vi "positionerCapture_example.vi"() -> ()   [LabVIEW 2023]
doc: "CONEX - CC Virtual Front Panel:\n\nThis is a sample of an application that can be built with the LabVIEW drivers.\n\nPress HOME / ENABLE in top left of panel to put stage in Ready state for motion."
uses:
  <vilib>/userDefined/High Color/IMAQdx.ctl
  <vilib>/Platform/TimedLoop/XDataNode/timing_clust.ctl
  <vilib>/Platform/TimedLoop/XDataNode/nitl_modes.ctl
  <vilib>/Platform/TimedLoop/XDataNode/wakeup.ctl
  <vilib>/Platform/TimedLoop/XDataNode/XDataNode.xnode
  <vilib>/Platform/TimedLoop/XDataNode/XDNodeRunTimeDep.lvlib
  <vilib>/vision/driver/NI_Vision_Acquisition_Software.lvlib
panel:
  in  "Session In":T1="BW14bits Focused"
  out "Current noUnits":dbl caption="mm" format="%#_6f"
  in  "lambda":dbl caption="nm" format="%#_6f"
  in  "Units":string(combo)="mm"
  in  "Go0":bool
  in  "Zero position":dbl caption="lam" format="%#_6f"
  in  "Tare":bool
  out "Relative position":dbl caption="lam" format="%#_6f"
  in  "Path to save the captures":path
  out "Image":T2(plugin-control)
  in  "(1) Go to:":dbl=1.0 caption="lam"
  out "Title":string
  in  "Set Max":bool
  in  "Set Min":bool
  in  "Max":dbl
  in  "Min":dbl
  in  "Set velocity":bool
  out "Stop cycle":bool=TRUE
  out "Title 2":string
  in  "Cycle":bool
  in  "Go2":bool
  in  "Go1":bool
  in  "(2) Go to:":dbl=1.0 caption="lam"
  in  "-":bool
  in  "+":bool
  in  "Step:":dbl caption="lam" format="%#_6f"
  out "Position History":dbl(graph)=1.5
  in  "Action":bool
  out "Stop polling":bool=TRUE
  out "Controller state description":string="STATUS"
  out "Velocity MAX":dbl=0.4
  out "Controller state":string="33"
  out "Positioner error":string="0000"
  in  "Velocity:":dbl format="%#_6f"
  in  "Exit":bool=TRUE
  out "Target position":dbl
  in  "Exit":bool
  in  "Position glissière":cluster{dbl, dbl}(slide) scale=0.0..25.0
  out "Current position":dbl caption="lam" format="%#_6f"
  # "mm/s"
  # "mm"
  # "Limits:"
  # "mm"
  # "(1)"
  # "(2)"
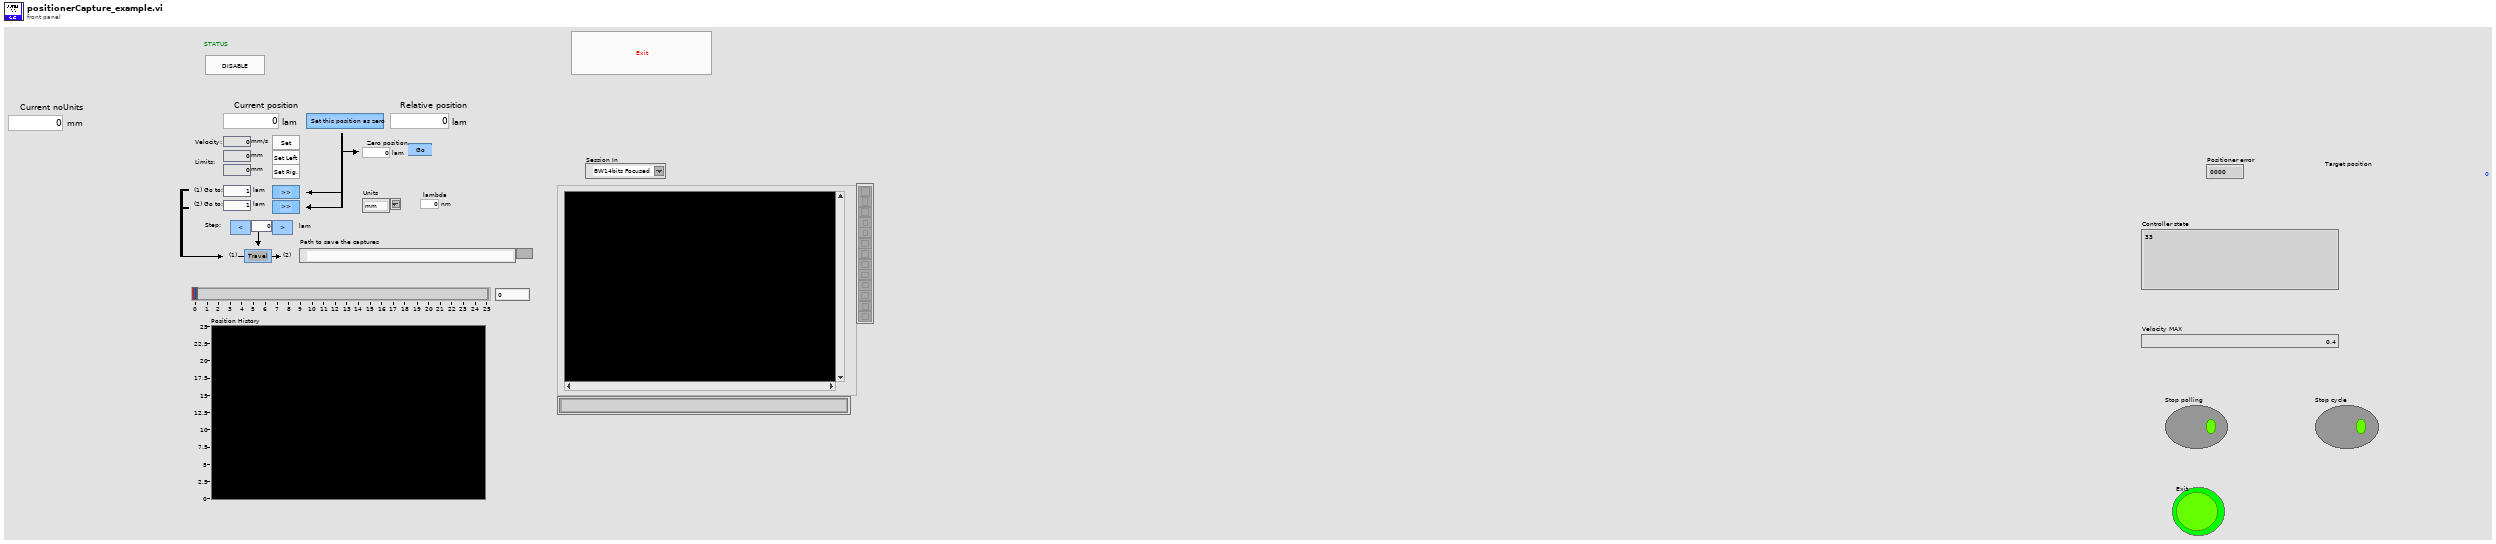
[diagram p1: front panel]
types:
  T1 = typedef "IMAQdx.ctl" = refnum<k21>
  T2 = typedef "IMAQ Image.ctl" = refnum<image>
  T3 = typedef "XDNodeRunTimeDep.lvlib/timing_clust.ctl" = cluster{"Expected End [f-1]":u64, "Actual End [f-1]":u64, "Finished Late? [f-1]":bool, "Expected End [i-1]":u64, "Actual End [i-1]":u64, "Finished Late? [i-1]":bool, "Expected Start [i]":u64, "Actual Start [i]":u64, "Expected Start [f]":u64, "Actual Start [f]":u64, "Source Name":string, "Structure Name":string, "Period":i64, "Deadline":i64, "Offset":i64, "Start":i64, "Priority":i32, "Timeout":i32, "Mode":T4, "Wakeup Reason":T5, "Error":errorcluster, "Source Type":string, "Secondary Source Type":string, "Global End Time":u64, "Global Start Time":u64, "Frame Duration":u64, "Iteration Duration":u64, "Assigned CPU":i32, "I/O Scan Engine Mode":u32}
  T4 = typedef "XDNodeRunTimeDep.lvlib/nitl_modes.ctl" = enum32{"No Change", "Process missed periods, maintain original phase", "Discard missed periods, maintain original phase", "Process missed periods, ignore original phase", "Discard missed periods, ignore original phase"}
  T5 = typedef "XDNodeRunTimeDep.lvlib/wakeup.ctl" = enum32{"Normal", "Aborted", "Asynchronous wakeup", "Timing source error", "Timed loop error", "Timeout"}
  T6 = cluster{"VISA resource name":refnum<visa-resource-name>, "Device name":string, "Controller address":i32, "error":errorcluster}
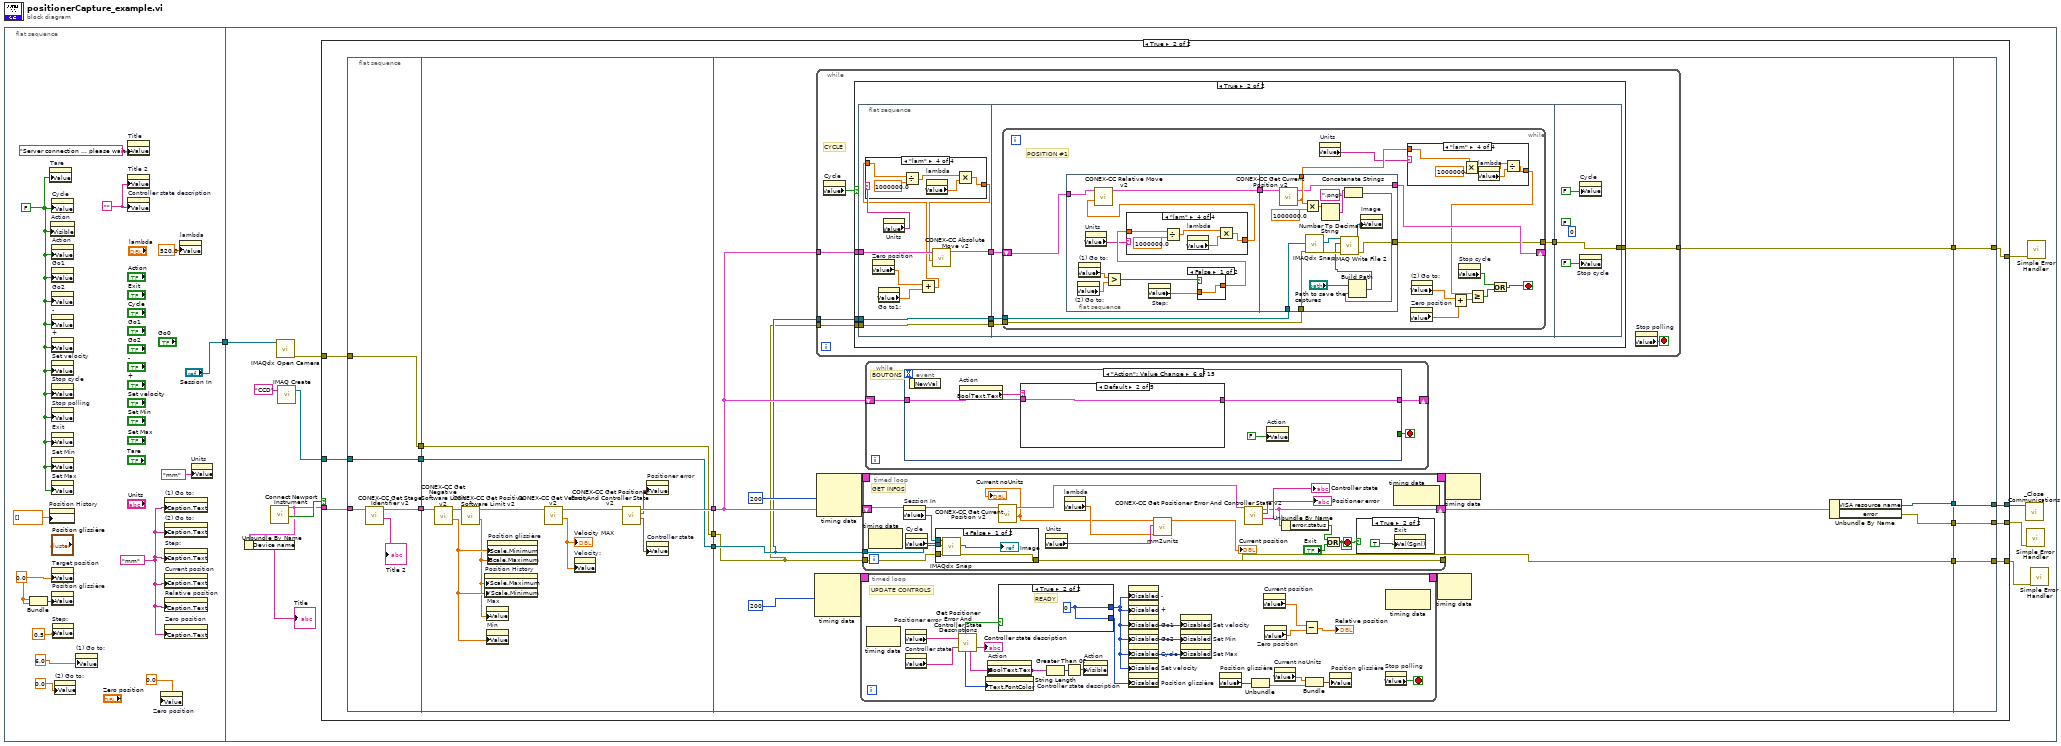
[diagram p0: block diagram]
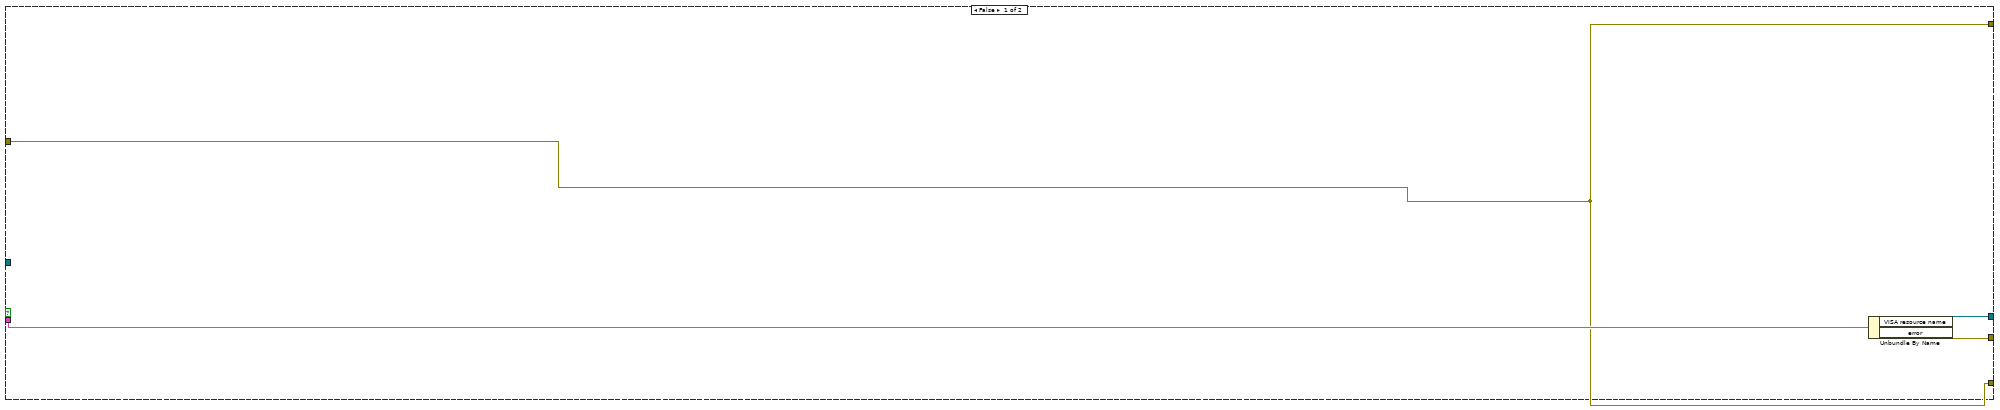
[diagram p2: hidden frame]
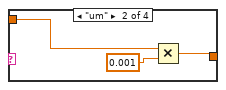
[diagram p5: hidden frame]
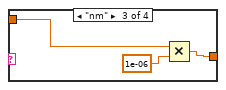
[diagram p6: hidden frame]
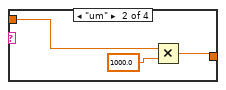
[diagram p8: hidden frame]
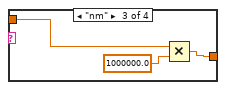
[diagram p9: hidden frame]
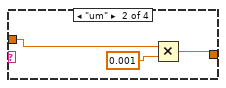
[diagram p11: hidden frame]
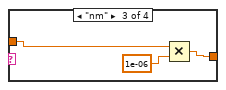
[diagram p12: hidden frame]
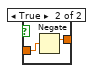
[diagram p13: hidden frame]
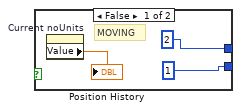
[diagram p14: hidden frame]
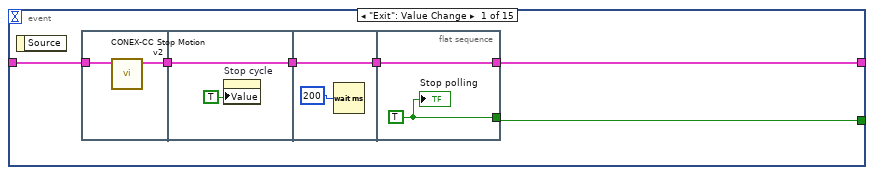
[diagram p15: hidden frame]
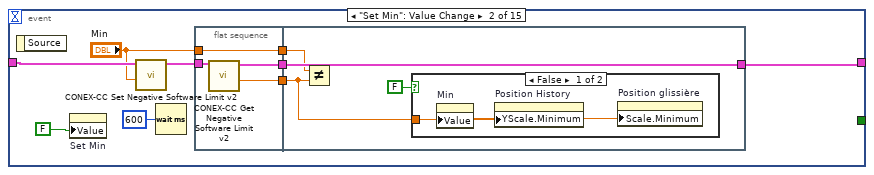
[diagram p16: hidden frame]
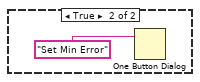
[diagram p17: hidden frame]
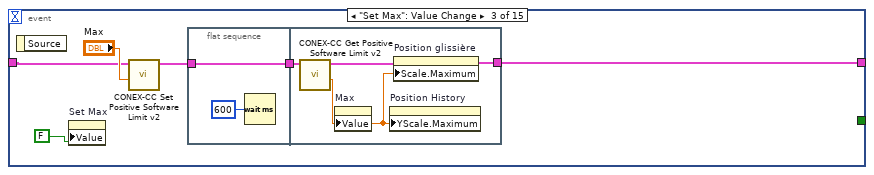
[diagram p18: hidden frame]
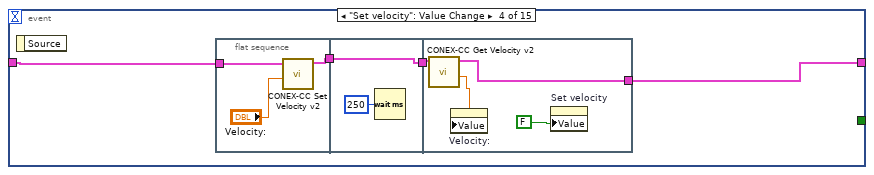
[diagram p19: hidden frame]
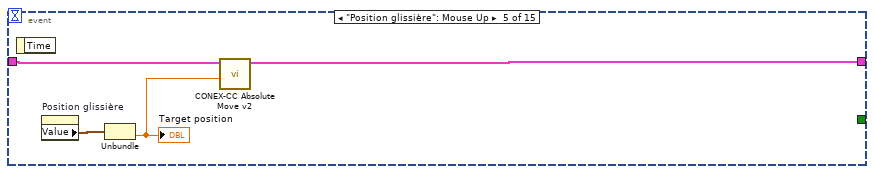
[diagram p20: hidden frame]
diagram:
  n1 = flat-sequence {
    tunnel: ["Session In"] -> w1
    tunnel: w1 -> [w16]
    frame #0 {
      w4 = "mm" ("Units")
      w8 = FALSE
      w14 = 0.0
      w13 = ""
      n2 = Bundle(w14, w14) -> (w15:cluster{dbl, dbl})  [unwired: 1 out]
      n3 = property on="Position History" class="WFChart (strict)"("History Data"=dbl[] [] ("Données d'historique")) -> ()  [unwired: 2 in, 2 out]
      n4 = property on="Tare" class="Bool (strict)"("Value"=w8) -> ()  [unwired: 2 in, 2 out]
      n5 = property on="Action" class="Bool (strict)"("Visible"=w8) -> ()  [unwired: 2 in, 2 out]
      n6 = property on="Cycle" class="Bool (strict)"("Value"=w8) -> ()  [unwired: 2 in, 2 out]
      n7 = property on="Action" class="Bool (strict)"("Value"=w8) -> ()  [unwired: 2 in, 2 out]
      n8 = property on="Go1" class="Bool (strict)"("Value"=w8) -> ()  [unwired: 2 in, 2 out]
      n9 = property on="Go2" class="Bool (strict)"("Value"=w8) -> ()  [unwired: 2 in, 2 out]
      n10 = property on="-" class="Bool (strict)"("Value"=w8) -> ()  [unwired: 2 in, 2 out]
      n11 = property on="+" class="Bool (strict)"("Value"=w8) -> ()  [unwired: 2 in, 2 out]
      n12 = property on="Set velocity" class="Bool (strict)"("Value"=w8) -> ()  [unwired: 2 in, 2 out]
      n13 = property on="Stop cycle" class="Bool (strict)"("Value"=w8) -> ()  [unwired: 2 in, 2 out]
      n14 = property on="Stop polling" class="Bool (strict)"("Value"=w8) -> ()  [unwired: 2 in, 2 out]
      n15 = property on="Exit" class="Bool (strict)"("Value"=w8) -> ()  [unwired: 2 in, 2 out]
      n16 = property on="Set Min" class="Bool (strict)"("Value"=w8) -> ()  [unwired: 2 in, 2 out]
      n17 = property on="Set Max" class="Bool (strict)"("Value"=w8) -> ()  [unwired: 2 in, 2 out]
      n18 = property on="Target position" class="DigNum (strict)"("Value"=w14) -> ()  [unwired: 2 in, 2 out]
      n19 = property on="Position glissière" class="Slide (strict)"("Value"=w15) -> ()  [unwired: 2 in, 2 out]
      n20 = property on="Step:" class="DigNum (strict)"("Value"=0.5 ("Step")) -> ()  [unwired: 2 in, 2 out]
      n21 = property on="(2) Go to:" class="DigNum (strict)"("Value"=0.0 ("Abs. Move 2")) -> ()  [unwired: 2 in, 2 out]
      n22 = property on="(1) Go to:" class="DigNum (strict)"("Value"=6.0 ("Abs. Move 1")) -> ()  [unwired: 2 in, 2 out]
      n23 = property on="Title" class="Str"("Value"="Server connection ... please wait." ("Title")) -> ()  [unwired: 2 in, 2 out]
      n24 = property on="Title 2" class="Str"("Value"=w13) -> ()  [unwired: 2 in, 2 out]
      n25 = property on="Controller state description" class="Str"("Value"=w13) -> ()  [unwired: 2 in, 2 out]
      n26 = property on="Zero position" class="DigNum (strict)"("Value"=0.0 ("Zero position")) -> ()  [unwired: 2 in, 2 out]
      n27 = property on="(1) Go to:" class="DigNum (strict)"("Caption.Text"=w4) -> ()  [unwired: 2 in, 2 out]
      n28 = property on="(2) Go to:" class="DigNum (strict)"("Caption.Text"=w4) -> ()  [unwired: 2 in, 2 out]
      n29 = property on="Step:" class="DigNum (strict)"("Caption.Text"=w4) -> ()  [unwired: 2 in, 2 out]
      n30 = property on="Current position" class="DigNum (strict)"("Caption.Text"=w4) -> ()  [unwired: 2 in, 2 out]
      n31 = property on="Relative position" class="DigNum (strict)"("Caption.Text"=w4) -> ()  [unwired: 2 in, 2 out]
      n32 = property on="Zero position" class="DigNum (strict)"("Caption.Text"=w4) -> ()  [unwired: 2 in, 2 out]
      n33 = property on="lambda" class="DigNum (strict)"("Value"=520.0 ("lambda")) -> ()  [unwired: 2 in, 2 out]
      n34 = property on="Units" class="CmbBox"("Value"="mm" ("Units")) -> ()  [unwired: 2 in, 2 out]
    }
    frame #1 {
      n35 = call "Connect Newport Instrument.vi"() -> ("Connected"=w24:bool, "Device Connection Cluster"=w23:T6)  [unwired: 6 in, 4 out]
      n36 = Unbundle By Name(w23) -> ("Device name"=→"Title":string)
      n37 = call <vilib>:"IMAQdx Open Camera.vi"("Session In"=w16) -> ("error out"=w19:errorcluster)  [unwired: 9 in, 1 out]
      n38 = call "IMAQ Create"("Image Name"="CCD") -> ("New Image"=w20:T2)  [unwired: 4 in, 1 out]
      n39 = case shown="True" w24 {
        tunnel: [w29 w47] -> w26
        tunnel: w23 -> [w30 w45]
        tunnel: [w28 w41] -> w22
        tunnel: w20 -> [_ w39]
        tunnel: w19 -> [w27 w36]
        tunnel: [w27 w33] -> w18
        tunnel: [w27 w31] -> w17
        frame False {
          n40 = Unbundle By Name(w30) -> ("VISA resource name"=w28:refnum<visa-resource-name>, "error"=w29:errorcluster)
        }
        frame True {
          n41 = flat-sequence {
            tunnel: w45 -> [w52]
            tunnel: [w50] -> w44
            tunnel: [w49] -> w40
            tunnel: w39 -> [w49]
            tunnel: [w48] -> w37
            tunnel: w36 -> [w48]
            tunnel: [w61] -> w46
            tunnel: w44 -> [w58]
            tunnel: w40 -> [w54]
            tunnel: [w54] -> w38
            tunnel: w37 -> [w53]
            tunnel: [w53] -> w35
            tunnel: w46 -> [w69]
            tunnel: [w71] -> w43
            tunnel: [w70] -> w42
            tunnel: w38 -> [w68]
            tunnel: w35 -> [w67]
            tunnel: [w66] -> w34
            tunnel: [w65] -> w32
            tunnel: [w453] -> w47
            tunnel: w43 -> [w452]
            tunnel: w42 -> [w453]
            tunnel: [w452] -> w41
            tunnel: [w451] -> w33
            tunnel: w34 -> [w451]
            tunnel: [w450] -> w31
            tunnel: w32 -> [w450]
            frame #0 {
              n42 = call "CONEX-CC Get Stage Identifier v2.vi"("Connection Cluster in"=w52) -> ("Identifier"=→"Title 2":string, "Connection Cluster out"=w50:T6)  [unwired: 9 in]
            }
            frame #1 {
              n43 = call "CONEX-CC Get Negative Software Limit v2.vi"("Connection Cluster in"=w58) -> ("Left limit"=w63:dbl, "Connection Cluster out"=w57:T6)  [unwired: 9 in]
              n44 = call "CONEX-CC Get Positive Software Limit v2.vi"("Connection Cluster in"=w57) -> ("Right limit"=w62:dbl, "Connection Cluster out"=w56:T6)  [unwired: 9 in]
              n45 = property on="Position History" class="WFChart (strict)"("YScale.Maximum"=w62, "YScale.Minimum"=w63) -> ()  [unwired: 2 in, 2 out]
              n46 = property on="Max" class="DigNum (strict)"("Value"=w62) -> ()  [unwired: 2 in, 2 out]
              n47 = property on="Min" class="DigNum (strict)"("Value"=w63) -> ()  [unwired: 2 in, 2 out]
              n48 = property on="Position glissière" class="Slide (strict)"("Scale.Minimum"=w63, "Scale.Maximum"=w62) -> ()  [unwired: 2 in, 2 out]
              n49 = call "CONEX-CC Get Velocity v2.vi"("Connection Cluster in"=w56) -> ("Velocity"=w64:dbl, "Connection Cluster out"=w55:T6)  [unwired: 8 in, 1 out]
              "Velocity MAX" <- w64
              n50 = property on="Velocity:" class="DigNum (strict)"("Value"=w64) -> ()  [unwired: 2 in, 2 out]
              n51 = call "CONEX-CC Get Positioner Error And Controller State v2.vi"("Connection Cluster in"=w55) -> ("Controller state"=w59:string, "Positioner error"=w60:string, "Connection Cluster out"=w61:T6)  [unwired: 8 in]
              n52 = property on="Positioner error" class="Str"("Value"=w60) -> ()  [unwired: 2 in, 2 out]
              n53 = property on="Controller state" class="Str"("Value"=w59) -> ()  [unwired: 2 in, 2 out]
            }
            frame #2 {
              n54 = node-c288(i64 200 ("Période")) -> (w76:T3)  [unwired: 1 in, 1 out]
              n55 = while {
                tunnel: w69 -> [w84]
                tunnel: w68 -> [w81]
                tunnel: w67 -> [w80]
                tunnel: [w79] -> w65
                stop <- w83 stop-if-true
                # "CYCLE"
                n56 = property on="Cycle" class="Bool (strict)"() -> ("Value"=w82:bool)  [unwired: 2 in, 2 out]
                n57 = case shown="True" w82 {
                  tunnel: w84 -> [_ w93]
                  tunnel: w81 -> [_ w90]
                  tunnel: w80 -> [w85 w88]
                  tunnel: [w85 w87] -> w79
                  frame False {
                  }
                  frame True {
                    n58 = flat-sequence {
                      tunnel: w93 -> [w102]
                      tunnel: [w101] -> w92
                      tunnel: [w100] -> w91
                      tunnel: w90 -> [w100]
                      tunnel: [w99] -> w89
                      tunnel: w88 -> [w99]
                      tunnel: w92 -> [w118]
                      tunnel: w91 -> [w117]
                      tunnel: w89 -> [w116]
                      tunnel: [w115] -> w86
                      tunnel: [w186] -> w87
                      tunnel: w86 -> [w186]
                      frame #0 {
                        n59 = property on="Zero position" class="DigNum (strict)"() -> ("Value"=w94:dbl)  [unwired: 2 in, 2 out]
                        n60 = property on="Go to1:" class="DigNum (strict)"() -> ("Value"=w96:dbl)  [unwired: 2 in, 2 out]
                        n61 = property on="Units" class="CmbBox"() -> ("Value"=w97:string)  [unwired: 2 in, 2 out]
                        n62 = Add(x=w94, y=w96) -> (x+y=w95:dbl)
                        n63 = case shown="\"lam\"" w97 {
                          tunnel: [w103 w104 w107 w110] -> w98
                          tunnel: w95 -> [w103 w105 w108 w114]
                          frame "mm", Default {
                          }
                          frame "um" {
                            n64 = Multiply(x=w105, y=0.001) -> (x*y=w104:dbl)
                          }
                          frame "nm" {
                            n65 = Multiply(x=w108, y=1e-06) -> (x*y=w107:dbl)
                          }
                          frame "lam" {
                            n66 = Divide(x=w114, y=1000000.0) -> (x/y=w112:dbl)
                            n67 = property on="lambda" class="DigNum (strict)"() -> ("Value"=w111:dbl)  [unwired: 2 in, 2 out]
                            n68 = Multiply(x=w112, y=w111) -> (x*y=w110:dbl)
                          }
                        }
                        n69 = call "CONEX-CC Absolute Move v2.vi"("Target position"=w98, "Connection Cluster in"=w102) -> ("Connection Cluster out"=w101:T6)  [unwired: 5 in, 2 out]
                      }
                      frame #1 {
                        n70 = while {
                          shift-right: [w127] -> _
                          shift-left: w118 -> [w132]
                          tunnel: w117 -> [w128]
                          tunnel: w116 -> [w129]
                          tunnel: [w126] -> w115
                          stop <- w133 stop-if-true
                          # "POSITION #1"
                          n71 = flat-sequence {
                            tunnel: w132 -> [w154]
                            tunnel: [w153] -> w125
                            tunnel: w128 -> [w185]
                            tunnel: w129 -> [w184]
                            tunnel: w125 -> [w180]
                            tunnel: [w172] -> w124
                            tunnel: [w171] -> w127
                            tunnel: [w170] -> w126
                            frame #0 {
                              n72 = property on="(2) Go to:" class="DigNum (strict)"() -> ("Value"=w152:dbl)  [unwired: 2 in, 2 out]
                              n73 = property on="(1) Go to:" class="DigNum (strict)"() -> ("Value"=w151:dbl)  [unwired: 2 in, 2 out]
                              n74 = property on="Units" class="CmbBox"() -> ("Value"=w146:string)  [unwired: 2 in, 2 out]
                              n75 = Greater?(x=w151, y=w152) -> (0:w150:bool)
                              n76 = property on="Step:" class="DigNum (strict)"() -> ("Value"=w149:dbl)  [unwired: 2 in, 2 out]
                              n77 = case shown="False" w150 {
                                tunnel: [w167 w168] -> w148
                                tunnel: w149 -> [w167 w169]
                                frame False {
                                }
                                frame True {
                                n78 = Negate(x=w169) -> (-x=w168:dbl)
                                }
                              }
                              n79 = case shown="\"lam\"" w146 {
                                tunnel: [w155 w157 w160 w163] -> w147
                                tunnel: w148 -> [w155 w156 w159 w162]
                                frame "mm", Default {
                                }
                                frame "um" {
                                n80 = Multiply(x=w156, y=0.001) -> (x*y=w157:dbl)
                                }
                                frame "nm" {
                                n81 = Multiply(x=w159, y=1e-06) -> (x*y=w160:dbl)
                                }
                                frame "lam" {
                                n82 = Divide(x=w162, y=1000000.0) -> (x/y=w165:dbl)
                                n83 = property on="lambda" class="DigNum (strict)"() -> ("Value"=w164:dbl)  [unwired: 2 in, 2 out]
                                n84 = Multiply(x=w165, y=w164) -> (x*y=w163:dbl)
                                }
                              }
                              n85 = call "CONEX-CC Relative Move v2.vi"("Relative displacement"=w147, "Connection Cluster in"=w154) -> ("Connection Cluster out"=w153:T6)  [unwired: 9 in]
                            }
                            frame #1 {
                              n86 = call "CONEX-CC Get Current Position v2.vi"("Connection Cluster in"=w180) -> ("Current position"=w172:dbl, "Connection Cluster out"=w171:T6)  [unwired: 8 in, 1 out]
                              n87 = Multiply(x=w172, y=1000000.0) -> (x*y=w176:dbl)
                              n88 = call <vilib>:"IMAQdx Snap.vi"("error in"=w184, "Image In"=w185) -> ("error out"=w182:errorcluster, "Image Out"=w183:T2)  [unwired: 7 in, 1 out]
                              n89 = Number To Decimal String(number=w176) -> (decimal integer string=w175:string)  [unwired: 1 in]
                              n90 = Concatenate Strings(w175, ".png" ("string")) -> (w173:string)
                              n91 = Build Path(base path="Path to save the captures", name or relative path=w173) -> (appended path=w177:path)
                              n92 = call-poly "IMAQ Write File 2"("error in (no error)"=w182, "File Path"=w177, "Image"=w183) -> ("error out"=w170:errorcluster, "Image Out (duplicate)"=w181:T2)  [unwired: 7 in]
                              n93 = property on="Image" class="ImageControl"("Value"=w181) -> ()  [unwired: 2 in, 2 out]
                            }
                          }
                          n94 = property on="Units" class="CmbBox"() -> ("Value"=w122:string)  [unwired: 2 in, 2 out]
                          n95 = case shown="\"lam\"" w122 {
                            tunnel: [w134 w135 w138 w141] -> w123
                            tunnel: w124 -> [w134 w136 w139 w142]
                            frame "mm", Default {
                            }
                            frame "um" {
                              n96 = Multiply(x=w136, y=1000.0) -> (x*y=w135:dbl)
                            }
                            frame "nm" {
                              n97 = Multiply(x=w139, y=1000000.0) -> (x*y=w138:dbl)
                            }
                            frame "lam" {
                              n98 = Multiply(x=w142, y=1000000.0) -> (x*y=w145:dbl)
                              n99 = property on="lambda" class="DigNum (strict)"() -> ("Value"=w143:dbl)  [unwired: 2 in, 2 out]
                              n100 = Divide(x=w145, y=w143) -> (x/y=w141:dbl)
                            }
                          }
                          n101 = property on="Zero position" class="DigNum (strict)"() -> ("Value"=w119:dbl)  [unwired: 2 in, 2 out]
                          n102 = property on="(2) Go to:" class="DigNum (strict)"() -> ("Value"=w120:dbl)  [unwired: 2 in, 2 out]
                          n103 = Add(x=w120, y=w119) -> (x+y=w121:dbl)
                          n104 = property on="Stop cycle" class="Bool (strict)"() -> ("Value"=w130:bool)  [unwired: 2 in, 2 out]
                          n105 = Greater Or Equal?(x=w123, y=w121) -> (x >= y?=w131:bool)
                          n106 = Or(x=w130, y=w131) -> (x .or. y?=w133:bool)
                        }
                      }
                      frame #2 {
                        (unwired) 0 ("counter")
                        (unwired) FALSE ("Visible")
                        n107 = property on="Cycle" class="Bool (strict)"("Value"=FALSE ("Cycle")) -> ()  [unwired: 2 in, 2 out]
                        n108 = property on="Stop cycle" class="Bool (strict)"("Value"=FALSE ("Cycle")) -> ()  [unwired: 2 in, 2 out]
                      }
                    }
                  }
                }
                n109 = property on="Stop polling" class="Bool (strict)"() -> ("Value"=w83:bool)  [unwired: 2 in, 2 out]
              }
              n110 = node-c288(i64 200 ("Période")) -> (w78:T3)  [unwired: 1 in, 1 out]
              n111 = timed-loop {
                timing: w76 -> [_]
                timing-out: [_] -> w75
                stop <- w197 stop-if-true
                # "UPDATE CONTROLS"
                n112 = node-c288() -> ()  [unwired: 2 out]
                n113 = property on="Positioner error" class="Str"() -> ("Value"=w206:string)  [unwired: 2 in, 2 out]
                n114 = property on="Controller state" class="Str"() -> ("Value"=w205:string)  [unwired: 2 in, 2 out]
                n115 = call "Get Positioner Error And Controller State Descriptions.vi"("Controller state"=w205, "Positioner error"=w206) -> ("Color"=w203:u32, "Action name"=w202:string, "Controller state description"=→"Controller state description":string, "IsReady?"=w199:bool)  [unwired: 2 out]
                n116 = property on="Controller state description" class="Str"("Text.FontColor"=w203) -> ()  [unwired: 2 in, 2 out]
                n117 = property on="Action" class="Bool (strict)"("BoolText.Text"=w202) -> ()  [unwired: 2 in, 2 out]
                n118 = case shown="True" w199 {
                  tunnel: [u8 2 w210] -> w196
                  tunnel: [u8 1 w210] -> w198
                  frame False {
                    # "MOVING"
                    n119 = property on="Current noUnits" class="DigNum (strict)"() -> ("Value"=→"Position History":dbl)  [unwired: 2 in, 2 out]
                  }
                  frame True {
                    w210 = u8 0
                    # "READY"
                  }
                }
                n120 = String Length(string=w202) -> (length=w201:i32)
                n121 = Greater Than 0?(x=w201) -> (x > 0?=w200:bool)
                n122 = property on="Action" class="Bool (strict)"("Visible"=w200) -> ()  [unwired: 2 in, 2 out]
                n123 = property on="-" class="Bool (strict)"("Disabled"=w196) -> ()  [unwired: 2 in, 2 out]
                n124 = property on="+" class="Bool (strict)"("Disabled"=w196) -> ()  [unwired: 2 in, 2 out]
                n125 = property on="Go1" class="Bool (strict)"("Disabled"=w196) -> ()  [unwired: 2 in, 2 out]
                n126 = property on="Go2" class="Bool (strict)"("Disabled"=w196) -> ()  [unwired: 2 in, 2 out]
                n127 = property on="Cycle" class="Bool (strict)"("Disabled"=w196) -> ()  [unwired: 2 in, 2 out]
                n128 = property on="Set velocity" class="Bool (strict)"("Disabled"=w196) -> ()  [unwired: 2 in, 2 out]
                n129 = property on="Position glissière" class="Slide (strict)"("Disabled"=w198) -> ()  [unwired: 2 in, 2 out]
                n130 = property on="Set velocity" class="Bool (strict)"("Disabled"=w196) -> ()  [unwired: 2 in, 2 out]
                n131 = property on="Set Min" class="Bool (strict)"("Disabled"=w196) -> ()  [unwired: 2 in, 2 out]
                n132 = property on="Set Max" class="Bool (strict)"("Disabled"=w196) -> ()  [unwired: 2 in, 2 out]
                n133 = property on="Position glissière" class="Slide (strict)"() -> ("Value"=w194:cluster{dbl, dbl})  [unwired: 2 in, 2 out]
                n134 = Unbundle(w194) -> (w193:dbl)  [unwired: 1 out]
                n135 = property on="Current position" class="DigNum (strict)"() -> ("Value"=w189:dbl)  [unwired: 2 in, 2 out]
                n136 = property on="Zero position" class="DigNum (strict)"() -> ("Value"=w190:dbl)  [unwired: 2 in, 2 out]
                n137 = property on="Current noUnits" class="DigNum (strict)"() -> ("Value"=w191:dbl)  [unwired: 2 in, 2 out]
                n138 = Subtract(x=w189, y=w190) -> (x-y=→"Relative position":dbl)
                n139 = Bundle("Value"=w191, w193) -> (w195:cluster{"Value":dbl, dbl})  [unwired: 1 out]
                n140 = property on="Position glissière" class="Slide (strict)"("Value"=w195) -> ()  [unwired: 2 in, 2 out]
                n141 = node-c288() -> ()  [unwired: 2 out]
                n142 = property on="Stop polling" class="Bool (strict)"() -> ("Value"=w197:bool)  [unwired: 2 in, 2 out]
              }
              n143 = timed-loop {
                timing: w78 -> [_]
                timing-out: [_] -> w77
                shift-right: [w427] -> w72
                shift-left: w69 -> [w436]
                tunnel: w68 -> [w435]
                tunnel: w67 -> [w434]
                tunnel: [w433] -> w66
                stop <- w430 stop-if-true
                # "GET INFOS"
                n144 = node-c288() -> ()  [unwired: 2 out]
                n145 = property on="Session In" class="IMAQdx (strict)"() -> ("Value"=w423:T1)  [unwired: 2 in, 2 out]
                n146 = property on="Cycle" class="Bool (strict)"() -> ("Value"=w432:bool)  [unwired: 2 in, 2 out]
                n147 = case shown="False" w432 {
                  tunnel: w435 -> [w441 _]
                  tunnel: w434 -> [w440 w442]
                  tunnel: [w438 w442] -> w433
                  tunnel: w423 -> [w437 _]
                  frame False {
                    n148 = call <vilib>:"IMAQdx Snap.vi"("error in"=w440, "Image In"=w441, "Session In"=w437) -> ("error out"=w438:errorcluster, "Image Out"=→"Image":T2)  [unwired: 6 in, 1 out]
                  }
                  frame True {
                  }
                }
                n149 = call "CONEX-CC Get Current Position v2.vi"("Connection Cluster in"=w436) -> ("Current position"=w420:dbl, "Connection Cluster out"=w424:T6)  [unwired: 8 in, 1 out]
                "Current noUnits" <- w420
                n150 = property on="Units" class="CmbBox"() -> ("Value"=w422:string)  [unwired: 2 in, 2 out]
                n151 = property on="lambda" class="DigNum (strict)"() -> ("Value"=w421:dbl)  [unwired: 2 in, 2 out]
                n152 = call "mm2units.vi"("lambda (nm)"=w421, "target units"=w422, "raw position (mm)"=w420) -> ("position in units"=→"Current position":dbl)  [unwired: 8 in]
                n153 = call "CONEX-CC Get Positioner Error And Controller State v2.vi"("Connection Cluster in"=w424) -> ("Controller state"=→"Controller state":string, "Positioner error"=→"Positioner error":string, "Connection Cluster out"=w427:T6)  [unwired: 8 in]
                n154 = Unbundle By Name(w427) -> ("error.status"=w425:bool)
                n155 = Or(x=w425, y="Exit") -> (x .or. y?=w430:bool)
                n156 = case shown="True" w430 {
                  frame False {
                  }
                  frame True {
                    n157 = property on="Exit" class="Bool (strict)"("Val(Sgnl)"=TRUE) -> ()  [unwired: 2 in, 2 out]
                  }
                }
                n158 = node-c288() -> ()  [unwired: 2 out]
              }
              n159 = while {
                shift-right: [w219] -> _
                shift-left: w69 -> [w218]
                stop <- w217 stop-if-true
                # "BOUTONS"
                n160 = event shown="[5] \"Action\": Value Change" {
                  selector: _ -> [_ _ _ _ _ _ _ _ _ _ _ _ _ _ _]
                  dyn-events: _ -> [_ _ _ _ _ _ _ _ _ _ _ _ _ _ _]
                  timeout: _ -> [_ _ _ _ _ _ _ _ _ _ _ _ _ _ _]
                  tunnel: [w223 _ _ _ _ _ _ _ _ _ _ _ _ _ _] -> w217
                  tunnel: w218 -> [w220 w240 w254 w267 w279 w283 w302 w323 w344 w364 w381 w397 w399 w408 _]
                  tunnel: [w225 w239 w253 w264 w278 w282 w301 w324 w343 w363 w382 w397 w399 w408 _] -> w219
                  event "Exit": Value Change {
                    n161 = event-data() -> ()  [unwired: 2 out]
                    n162 = flat-sequence {
                      tunnel: [w227] -> w224
                      tunnel: w220 -> [w226]
                      tunnel: w224 -> [w229]
                      tunnel: [w229] -> w222
                      tunnel: w222 -> [w231]
                      tunnel: [w231] -> w221
                      tunnel: [w233] -> w225
                      tunnel: w221 -> [w233]
                      tunnel: [w232] -> w223
                      frame #0 {
                        n163 = call "CONEX-CC Stop Motion v2.vi"("Connection Cluster in"=w226) -> ("Connection Cluster out"=w227:T6)  [unwired: 10 in]
                      }
                      frame #1 {
                        n164 = property on="Stop cycle" class="Bool (strict)"("Value"=TRUE) -> ()  [unwired: 2 in, 2 out]
                      }
                      frame #2 {
                        n165 = Wait (ms)(milliseconds to wait=u32 200 ("attente (ms)")) -> ()  [unwired: 1 out]
                      }
                      frame #3 {
                        w232 = TRUE
                        "Stop polling" <- w232
                      }
                    }
                  }
                  event "Set Min": Value Change {
                    n166 = event-data() -> ()  [unwired: 2 out]
                    n167 = property on="Set Min" class="Bool (strict)"("Value"=FALSE ("Set Min")) -> ()  [unwired: 2 in, 2 out]
                    n168 = call "CONEX-CC Set Negative Software Limit v2.vi"("Negative limit (left)"="Min", "Connection Cluster in"=w240) -> ("Connection Cluster out"=w242:T6)  [unwired: 9 in]
                    n169 = Wait (ms)(milliseconds to wait=u32 600 ("attente (ms)")) -> ()  [unwired: 1 out]
                    n170 = flat-sequence {
                      tunnel: w242 -> [w246]
                      tunnel: [w245] -> w237
                      tunnel: [w244] -> w236
                      tunnel: "Min" -> [w244]
                      tunnel: [w243] -> w234
                      tunnel: [w250] -> w239
                      tunnel: w237 -> [w250]
                      tunnel: w236 -> [w249]
                      tunnel: w234 -> [w247]
                      frame #0 {
                        n171 = call "CONEX-CC Get Negative Software Limit v2.vi"("Connection Cluster in"=w246) -> ("Left limit"=w243:dbl, "Connection Cluster out"=w245:T6)  [unwired: 9 in]
                      }
                      frame #1 {
                        n172 = Not Equal?(x=w249, y=w247) -> ()  [unwired: 1 out]
                        n173 = case shown="False" FALSE {
                          tunnel: w247 -> [w251 _]
                          frame False {
                            n174 = property on="Min" class="DigNum (strict)"("Value"=w251) -> ()  [unwired: 2 in, 2 out]
                            n175 = property on="Position History" class="WFChart (strict)"("YScale.Minimum"=w251) -> ()  [unwired: 2 in, 2 out]
                            n176 = property on="Position glissière" class="Slide (strict)"("Scale.Minimum"=w251) -> ()  [unwired: 2 in, 2 out]
                          }
                          frame True {
                            n177 = One Button Dialog(message="Set Min Error") -> ()  [unwired: 1 in, 1 out]
                          }
                        }
                      }
                    }
                  }
                  event "Set Max": Value Change {
                    n178 = event-data() -> ()  [unwired: 2 out]
                    n179 = property on="Set Max" class="Bool (strict)"("Value"=FALSE ("Set Max")) -> ()  [unwired: 2 in, 2 out]
                    n180 = call "CONEX-CC Set Positive Software Limit v2.vi"("Positive limit (right)"="Max", "Connection Cluster in"=w254) -> ("Connection Cluster out"=w258:T6)  [unwired: 9 in]
                    n181 = flat-sequence {
                      tunnel: w258 -> [w260]
                      tunnel: [w260] -> w255
                      tunnel: [w263] -> w253
                      tunnel: w255 -> [w261]
                      frame #0 {
                        n182 = Wait (ms)(milliseconds to wait=u32 600 ("attente (ms)")) -> ()  [unwired: 1 out]
                      }
                      frame #1 {
                        n183 = call "CONEX-CC Get Positive Software Limit v2.vi"("Connection Cluster in"=w261) -> ("Right limit"=w262:dbl, "Connection Cluster out"=w263:T6)  [unwired: 9 in]
                        n184 = property on="Max" class="DigNum (strict)"("Value"=w262) -> ()  [unwired: 2 in, 2 out]
                        n185 = property on="Position History" class="WFChart (strict)"("YScale.Maximum"=w262) -> ()  [unwired: 2 in, 2 out]
                        n186 = property on="Position glissière" class="Slide (strict)"("Scale.Maximum"=w262) -> ()  [unwired: 2 in, 2 out]
                      }
                    }
                  }
                  event "Set velocity": Value Change {
                    n187 = event-data() -> ()  [unwired: 2 out]
                    n188 = flat-sequence {
                      tunnel: w267 -> [w269]
                      tunnel: [w268] -> w265
                      tunnel: [w272] -> w266
                      tunnel: w265 -> [w272]
                      tunnel: w266 -> [w276]
                      tunnel: [w275] -> w264
                      frame #0 {
                        n189 = call "CONEX-CC Set Velocity v2.vi"("Velocity"="Velocity:", "Connection Cluster in"=w269) -> ("Connection Cluster out"=w268:T6)  [unwired: 9 in]
                      }
                      frame #1 {
                        n190 = Wait (ms)(milliseconds to wait=u32 250 ("attente (ms)")) -> ()  [unwired: 1 out]
                      }
                      frame #2 {
                        n191 = call "CONEX-CC Get Velocity v2.vi"("Connection Cluster in"=w276) -> ("Velocity"=w274:dbl, "Connection Cluster out"=w275:T6)  [unwired: 8 in, 1 out]
                        n192 = property on="Velocity:" class="DigNum (strict)"("Value"=w274) -> ()  [unwired: 2 in, 2 out]
                        n193 = property on="Set velocity" class="Bool (strict)"("Value"=FALSE ("Set velocity")) -> ()  [unwired: 2 in, 2 out]
                      }
                    }
                  }
                  event "Position glissière": Mouse Up {
                    n194 = event-data() -> ()  [unwired: 2 out]
                    n195 = property on="Position glissière" class="Slide (strict)"() -> ("Value"=w280:cluster{dbl, dbl})  [unwired: 2 in, 2 out]
                    n196 = Unbundle(w280) -> (w277:dbl)  [unwired: 1 out]
                    "Target position" <- w277
                    n197 = call "CONEX-CC Absolute Move v2.vi"("Target position"=w277, "Connection Cluster in"=w279) -> ("Connection Cluster out"=w278:T6)  [unwired: 5 in, 2 out]
                  }
                  event "Action": Value Change {
                    n198 = event-data() -> ()  [unwired: 2 out]
                    n199 = property on="Action" class="Bool (strict)"() -> ("BoolText.Text"=w284:string)  [unwired: 2 in, 2 out]
                    n200 = case shown="Default" w284 {
                      tunnel: w283 -> [w286 w288 w290 w296 w298]
                      tunnel: [w285 w288 w289 w295 w300] -> w282
                      frame "ENABLE" {
                        n201 = call "CONEX-CC Enter-Leave DISABLE State v2.vi"("Ready? (false=DISABLE true=READY)"=TRUE ("Flag (false=DISABLE true=READY)"), "Connection Cluster in"=w286) -> ("Connection Cluster out"=w285:T6)  [unwired: 7 in]
                      }
                      frame Default {
                      }
                      frame "HOME" {
                        n202 = flat-sequence {
                          tunnel: w290 -> [w293]
                          tunnel: [w292] -> w289
                          frame #0 {
                            n203 = One Button Dialog(message="The Stage will go to the 0 position. Check that the travel is clean!") -> ()  [unwired: 1 in, 1 out]
                          }
                          frame #1 {
                            n204 = call "CONEX-CC Home search v2.vi"("Connection Cluster in"=w293) -> ("Connection Cluster out"=w292:T6)  [unwired: 5 in, 3 out]
                          }
                        }
                      }
                      frame "DISABLE" {
                        n205 = call "CONEX-CC Enter-Leave DISABLE State v2.vi"("Ready? (false=DISABLE true=READY)"=FALSE ("Flag (false=DISABLE true=READY)"), "Connection Cluster in"=w296) -> ("Connection Cluster out"=w295:T6)  [unwired: 7 in]
                      }
                      frame "STOP" {
                        n206 = call "CONEX-CC Stop Motion v2.vi"("Connection Cluster in"=w298) -> ("Connection Cluster out"=w300:T6)  [unwired: 10 in]
                        n207 = property on="Stop cycle" class="Bool (strict)"("Value"=TRUE) -> ()  [unwired: 2 in, 2 out]
                        "Stop cycle" <- TRUE ("Stop cycle")
                      }
                    }
                    n208 = property on="Action" class="Bool (strict)"("Value"=FALSE) -> ()  [unwired: 2 in, 2 out]
                  }
                  event "-": Value Change {
                    n209 = event-data() -> ()  [unwired: 2 out]
                    n210 = property on="-" class="Bool (strict)"("Value"=FALSE ("-")) -> ()  [unwired: 2 in, 2 out]
                    n211 = Negate(x="Step:") -> (-x=w305:dbl)
                    n212 = property on="Units" class="CmbBox"() -> ("Value"=w303:string)  [unwired: 2 in, 2 out]
                    n213 = case shown="\"lam\"" w303 {
                      tunnel: [w308 w309 w312 w315] -> w304
                      tunnel: w305 -> [w308 w310 w313 w319]
                      frame "mm", Default {
                      }
                      frame "um" {
                        n214 = Multiply(x=w310, y=0.001) -> (x*y=w309:dbl)
                      }
                      frame "nm" {
                        n215 = Multiply(x=w313, y=1e-06) -> (x*y=w312:dbl)
                      }
                      frame "lam" {
                        n216 = Divide(x=w319, y=1000000.0) -> (x/y=w317:dbl)
                        n217 = property on="lambda" class="DigNum (strict)"() -> ("Value"=w316:dbl)  [unwired: 2 in, 2 out]
                        n218 = Multiply(x=w317, y=w316) -> (x*y=w315:dbl)
                      }
                    }
                    n219 = call "CONEX-CC Relative Move v2.vi"("Relative displacement"=w304, "Connection Cluster in"=w302) -> ("Connection Cluster out"=w301:T6)  [unwired: 9 in]
                  }
                  event "+": Value Change {
                    n220 = event-data() -> ()  [unwired: 2 out]
                    n221 = property on="+" class="Bool (strict)"("Value"=FALSE ("+")) -> ()  [unwired: 2 in, 2 out]
                    n222 = property on="Step:" class="DigNum (strict)"() -> ("Value"=w322:dbl)  [unwired: 2 in, 2 out]
                    n223 = property on="Units" class="CmbBox"() -> ("Value"=w321:string)  [unwired: 2 in, 2 out]
                    n224 = case shown="\"lam\"" w321 {
                      tunnel: [w326 w327 w330 w333] -> w320
                      tunnel: w322 -> [w326 w328 w331 w337]
                      frame "mm", Default {
                      }
                      frame "um" {
                        n225 = Multiply(x=w328, y=0.001) -> (x*y=w327:dbl)
                      }
                      frame "nm" {
                        n226 = Multiply(x=w331, y=1e-06) -> (x*y=w330:dbl)
                      }
                      frame "lam" {
                        n227 = Divide(x=w337, y=1000000.0) -> (x/y=w335:dbl)
                        n228 = property on="lambda" class="DigNum (strict)"() -> ("Value"=w334:dbl)  [unwired: 2 in, 2 out]
                        n229 = Multiply(x=w335, y=w334) -> (x*y=w333:dbl)
                      }
                    }
                    n230 = call "CONEX-CC Relative Move v2.vi"("Relative displacement"=w320, "Connection Cluster in"=w323) -> ("Connection Cluster out"=w324:T6)  [unwired: 9 in]
                  }
                  event "Go1": Value Change {
                    n231 = event-data() -> ()  [unwired: 2 out]
                    n232 = property on="Go1" class="Bool (strict)"("Value"=FALSE ("Go1")) -> ()  [unwired: 2 in, 2 out]
                    n233 = property on="Zero position" class="DigNum (strict)"() -> ("Value"=w341:dbl)  [unwired: 2 in, 2 out]
                    n234 = property on="Units" class="CmbBox"() -> ("Value"=w342:string)  [unwired: 2 in, 2 out]
                    n235 = Add(x="(1) Go to:", y=w341) -> (x+y=w339:dbl)
                    n236 = case shown="\"lam\"" w342 {
                      tunnel: [w346 w347 w350 w353] -> w338
                      tunnel: w339 -> [w346 w348 w351 w357]
                      frame "mm", Default {
                      }
                      frame "um" {
                        n237 = Multiply(x=w348, y=0.001) -> (x*y=w347:dbl)
                      }
                      frame "nm" {
                        n238 = Multiply(x=w351, y=1e-06) -> (x*y=w350:dbl)
                      }
                      frame "lam" {
                        n239 = Divide(x=w357, y=1000000.0) -> (x/y=w355:dbl)
                        n240 = property on="lambda" class="DigNum (strict)"() -> ("Value"=w354:dbl)  [unwired: 2 in, 2 out]
                        n241 = Multiply(x=w355, y=w354) -> (x*y=w353:dbl)
                      }
                    }
                    n242 = call "CONEX-CC Absolute Move v2.vi"("Target position"=w338, "Connection Cluster in"=w344) -> ("Connection Cluster out"=w343:T6)  [unwired: 5 in, 2 out]
                  }
                  event "Go2": Value Change {
                    n243 = event-data() -> ()  [unwired: 2 out]
                    n244 = property on="Go2" class="Bool (strict)"("Value"=FALSE ("Go2")) -> ()  [unwired: 2 in, 2 out]
                    n245 = property on="Zero position" class="DigNum (strict)"() -> ("Value"=w361:dbl)  [unwired: 2 in, 2 out]
                    n246 = property on="Units" class="CmbBox"() -> ("Value"=w362:string)  [unwired: 2 in, 2 out]
                    n247 = Add(x="(2) Go to:", y=w361) -> (x+y=w359:dbl)
                    n248 = case shown="\"lam\"" w362 {
                      tunnel: [w366 w368 w371 w374] -> w358
                      tunnel: w359 -> [w366 w367 w370 w373]
                      frame "mm", Default {
                      }
                      frame "um" {
                        n249 = Multiply(x=w367, y=0.001) -> (x*y=w368:dbl)
                      }
                      frame "nm" {
                        n250 = Multiply(x=w370, y=1e-06) -> (x*y=w371:dbl)
                      }
                      frame "lam" {
                        n251 = Divide(x=w373, y=1000000.0) -> (x/y=w376:dbl)
                        n252 = property on="lambda" class="DigNum (strict)"() -> ("Value"=w375:dbl)  [unwired: 2 in, 2 out]
                        n253 = Multiply(x=w376, y=w375) -> (x*y=w374:dbl)
                      }
                    }
                    n254 = call "CONEX-CC Absolute Move v2.vi"("Target position"=w358, "Connection Cluster in"=w364) -> ("Connection Cluster out"=w363:T6)  [unwired: 5 in, 2 out]
                  }
                  event "Go0": Value Change {
                    n255 = event-data() -> ()  [unwired: 2 out]
                    n256 = property on="Zero position" class="DigNum (strict)"() -> ("Value"=w378:dbl)  [unwired: 2 in, 2 out]
                    n257 = property on="Go0" class="Bool (strict)"("Value"=FALSE ("Go2")) -> ()  [unwired: 2 in, 2 out]
                    n258 = property on="Units" class="CmbBox"() -> ("Value"=w379:string)  [unwired: 2 in, 2 out]
                    n259 = case shown="\"lam\"" w379 {
                      tunnel: [w384 w386 w389 w392] -> w380
                      tunnel: w378 -> [w384 w385 w388 w391]
                      frame "mm", Default {
                      }
                      frame "um" {
                        n260 = Multiply(x=w385, y=0.001) -> (x*y=w386:dbl)
                      }
                      frame "nm" {
                        n261 = Multiply(x=w388, y=1e-06) -> (x*y=w389:dbl)
                      }
                      frame "lam" {
                        n262 = Divide(x=w391, y=1000000.0) -> (x/y=w394:dbl)
                        n263 = property on="lambda" class="DigNum (strict)"() -> ("Value"=w393:dbl)  [unwired: 2 in, 2 out]
                        n264 = Multiply(x=w394, y=w393) -> (x*y=w392:dbl)
                      }
                    }
                    n265 = call "CONEX-CC Absolute Move v2.vi"("Target position"=w380, "Connection Cluster in"=w381) -> ("Connection Cluster out"=w382:T6)  [unwired: 5 in, 2 out]
                  }
                  event "Tare": Value Change {
                    n266 = event-data() -> ()  [unwired: 2 out]
                    n267 = property on="Tare" class="Bool (strict)"("Value"=FALSE ("Tare")) -> ()  [unwired: 2 in, 2 out]
                    n268 = property on="Current position" class="DigNum (strict)"() -> ("Value"=w396:dbl)  [unwired: 2 in, 2 out]
                    n269 = property on="Zero position" class="DigNum (strict)"("Value"=w396) -> ()  [unwired: 2 in, 2 out]
                  }
                  event "Cycle": Value Change {
                    (unwired) 0 ("Numérique")
                    n270 = event-data() -> ()  [unwired: 2 out]
                    n271 = property on="Cycle" class="Bool (strict)"("Value"=TRUE ("Cycle")) -> ()  [unwired: 2 in, 2 out]
                  }
                  event "Units": Value Change {
                    n272 = event-data() -> ("NewVal"=w407:string, "OldVal"=w406:string)  [unwired: 1 out]
                    n273 = property on="(1) Go to:" class="DigNum (strict)"("Caption.Text"=w407) -> ()  [unwired: 2 in, 2 out]
                    n274 = property on="(2) Go to:" class="DigNum (strict)"("Caption.Text"=w407) -> ()  [unwired: 2 in, 2 out]
                    n275 = property on="Step:" class="DigNum (strict)"("Caption.Text"=w407) -> ()  [unwired: 2 in, 2 out]
                    n276 = property on="Current position" class="DigNum (strict)"("Caption.Text"=w407) -> ()  [unwired: 2 in, 2 out]
                    n277 = property on="Relative position" class="DigNum (strict)"("Caption.Text"=w407) -> ()  [unwired: 2 in, 2 out]
                    n278 = property on="Zero position" class="DigNum (strict)"("Caption.Text"=w407) -> ()  [unwired: 2 in, 2 out]
                    n279 = case shown="\"mm\", Default" w406 {
                      tunnel: [1000000.0 ("y") 1000.0 ("y") 1.0 ("y") w412] -> w405
                      frame "mm", Default {
                      }
                      frame "um" {
                      }
                      frame "nm" {
                      }
                      frame "lam" {
                        n280 = property on="lambda" class="DigNum (strict)"() -> ("Value"=w412:dbl)  [unwired: 2 in, 2 out]
                      }
                    }
                    n281 = case shown="\"lam\"" w407 {
                      tunnel: [1000000.0 ("y") 1000.0 ("y") 1.0 ("y") w416] -> w404
                      frame "mm", Default {
                      }
                      frame "um" {
                      }
                      frame "nm" {
                      }
                      frame "lam" {
                        n282 = property on="lambda" class="DigNum (strict)"() -> ("Value"=w416:dbl)  [unwired: 2 in, 2 out]
                      }
                    }
                    n283 = property on="Zero position" class="DigNum (strict)"() -> ("Value"=w402:dbl)  [unwired: 2 in, 2 out]
                    n284 = Divide(x=w405, y=w404) -> (x/y=w403:dbl)
                    n285 = Multiply(x=w402, y=w403) -> (x*y=w401:dbl)
                    n286 = property on="Zero position" class="DigNum (strict)"("Value"=w401) -> ()  [unwired: 2 in, 2 out]
                  }
                  event Value Change {
                    n287 = event-data() -> ("OldVal"=w417:T1, "NewVal"=w419:T1)  [unwired: 5 out]
                    n288 = call <vilib>:"IMAQdx Close Camera.vi"("Session In"=w417) -> ()  [unwired: 10 in, 1 out]
                    n289 = call <vilib>:"IMAQdx Open Camera.vi"("Session In"=w419) -> ("Session Out"=w418:T1)  [unwired: 9 in, 1 out]
                    n290 = property on="Session In" class="IMAQdx (strict)"("Value"=w418) -> ()  [unwired: 2 in, 2 out]
                  }
                }
              }
              n291 = node-c288(w75) -> ()  [unwired: 1 out]
              n292 = node-c288(w77) -> ()  [unwired: 1 out]
              n293 = Unbundle By Name(w72) -> ("VISA resource name"=w71:refnum<visa-resource-name>, "error"=w70:errorcluster)
            }
            frame #3 {
            }
          }
        }
      }
      n294 = call "_Close Communications.vi"("Instrument Channel"=w22) -> ()  [unwired: 14 in, 1 out]
      n295 = call <vilib>:"Simple Error Handler.vi"("error in (no error)"=w26) -> ()  [unwired: 1 in, 8 out]
      n296 = call <vilib>:"Simple Error Handler.vi"("error in (no error)"=w17) -> ()  [unwired: 1 in, 8 out]
      n297 = call <vilib>:"Simple Error Handler.vi"("error in (no error)"=w18) -> ()  [unwired: 1 in, 8 out]
    }
  }
